vi "Time Out.vi"(11 "Timer DVR":refnum<data-value>) -> ()   [LabVIEW 2018, in "Timer.lvclass"]
uses:
  Timer.lvclass
  Timer.lvclass/Timer.ctl
  Get Target Time Elapsed Event.vi
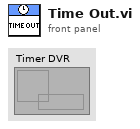
[diagram p1: front panel]
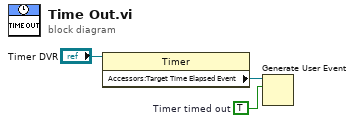
[diagram p0: block diagram]
diagram:
  w1 = TRUE  # Timer timed out
  n1 = property class="Timer"(reference="Timer DVR") -> ("Accessors:Target Time Elapsed Event"=w2:refnum<user-event>)  [unwired: 1 in, 2 out]
  n2 = Generate User Event(user event=w2, event data cluster=w1) -> ()  [unwired: 2 in, 2 out]
